vi "Task 4.vi"() -> ()   [LabVIEW 2025]
uses:
  <vilib>/httpClient/POSTBuffer.vi
  <vilib>/httpClient/LabVIEWHTTPClient.lvlib
panel:
  out "Corrected Text":string
  in  "Select correct word":string(combo)
  out "Error Text underlined":string
  in  "?":bool
  in  "User Input":string
  # "Users can check spelling inside a text box. Misspelled words are underlined, and users can select the correct suggestion to replace the incorrect word."
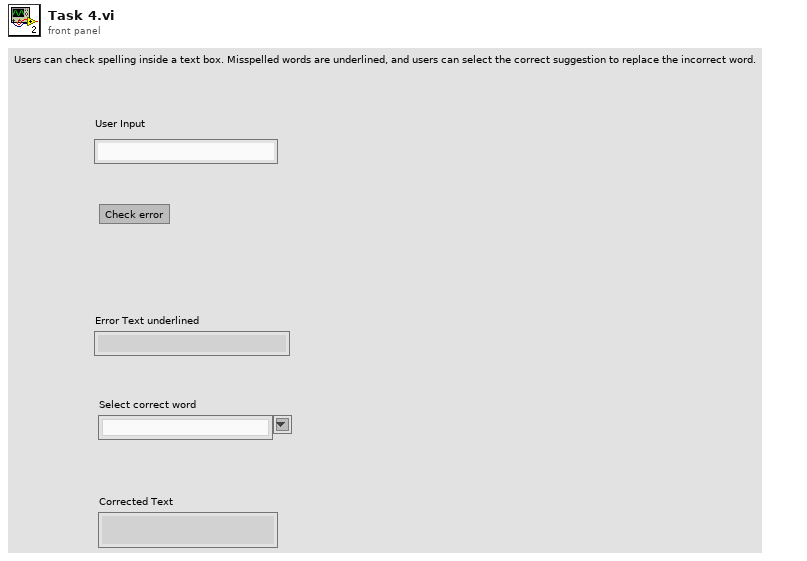
[diagram p1: front panel]
types:
  T1 = cluster{"matches":cluster{"offset":i32, "length":i32, "message":string, "replacements":cluster{"value":string}[]}[]}
  T2 = typedef "LabVIEWHTTPClient.lvlib/ClientHandle.ctl" = refnum<k1>
  T3 = cluster{"offset":i32, "length":i32, "message":string, "replacements":cluster{"value":string}[]}[]
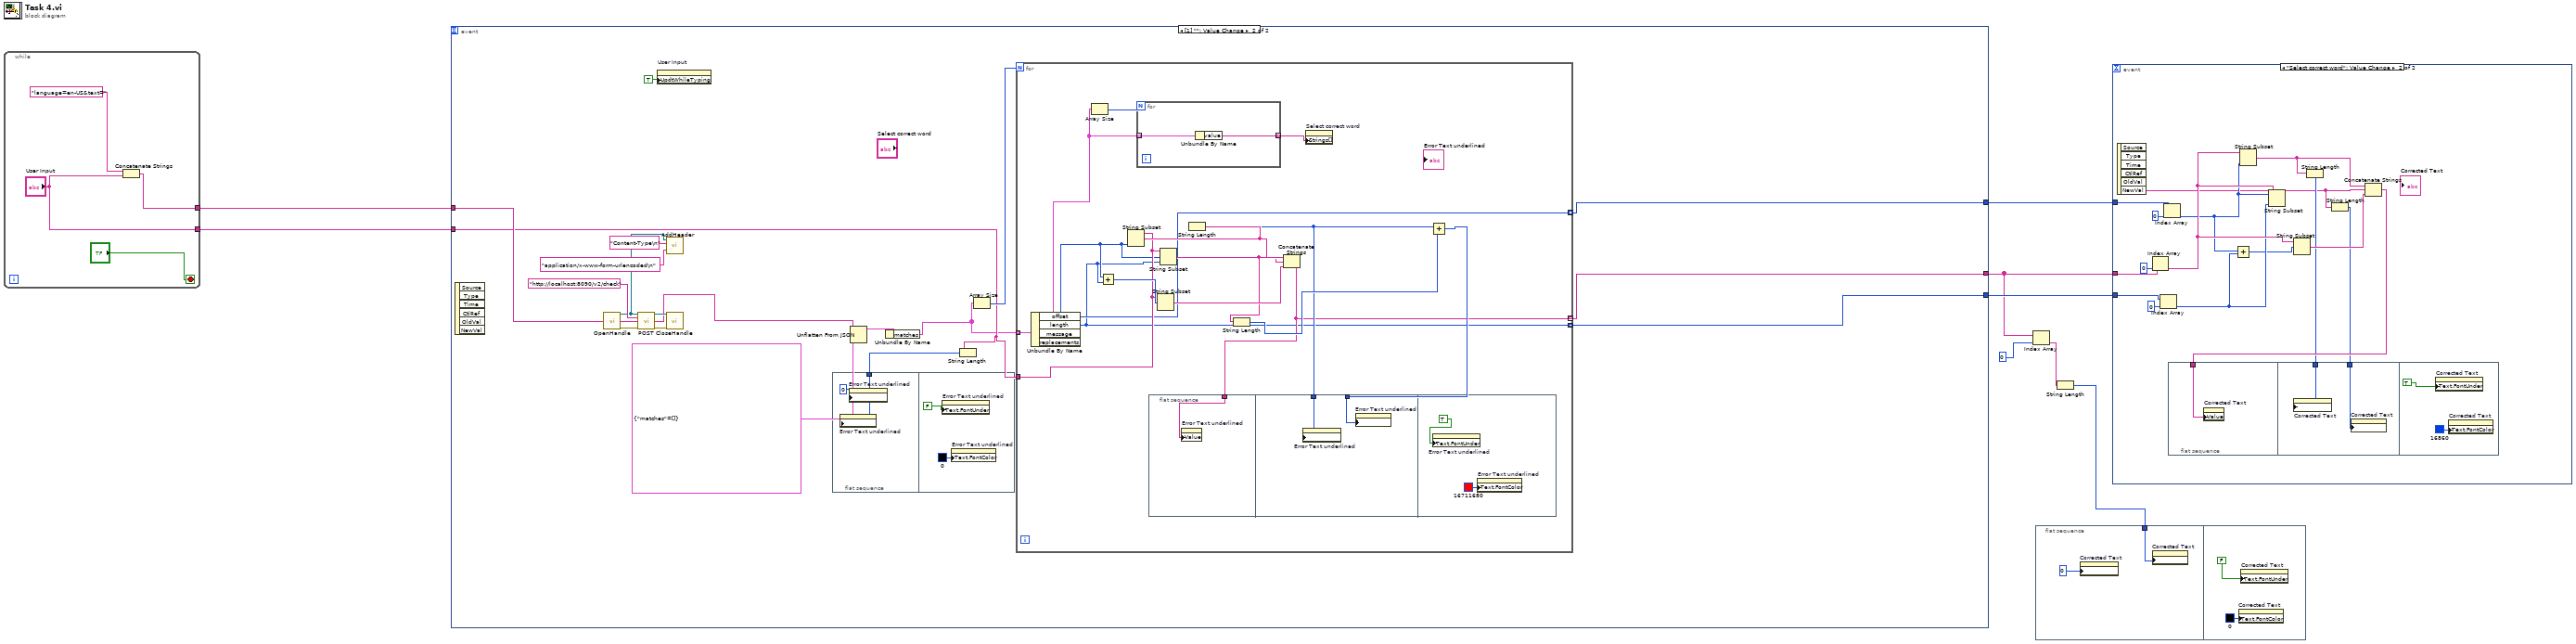
[diagram p0: block diagram]
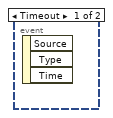
[diagram p2: hidden frame]
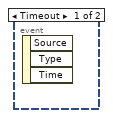
[diagram p3: hidden frame]
diagram:
  n1 = while {
    tunnel: ["User Input"] -> w2
    tunnel: [w10] -> w1
    stop <- "?" stop-if-true
    n2 = Concatenate Strings("language=en-US&text=", "User Input") -> (w10:string)
  }
  n3 = event shown="[1] \"\": Value Change" {
    selector: _ -> [_ _]
    dyn-events: _ -> [_ _]
    timeout: _ -> [_ _]
    tunnel: w1 -> [_ w24]
    tunnel: w2 -> [_ w19]
    tunnel: [_ w16] -> w8
    tunnel: [_ w15] -> w5
    tunnel: [_ w14] -> w7
    event Timeout {
      n4 = event-data() -> ()  [unwired: 1 in, 3 out]
    }
    event Value Change {
      n5 = event-data() -> ()  [unwired: 1 in, 6 out]
      n6 = call <vilib>:"OpenHandle.vi"() -> ("client handle out"=w27:T2, "error out"=w28:errorcluster)  [unwired: 14 in]
      n7 = call-poly <vilib>:"POST.vi"("client handle"=w27, "url"="http://localhost:8090/v2/check", "buffer"=w24, "error in (no error)"=w28) -> ("client handle out"=w30:T2, "body"=w23:string, "error out"=w29:errorcluster)  [unwired: 8 in, 1 out]
      n8 = property on="User Input" class="Str"("UpdtWhileTyping"=TRUE ("Update While Typing?")) -> ()  [unwired: 2 in, 2 out]
      n9 = call <vilib>:"AddHeader.vi"("client handle"=w27, "header"="Content-Type\n", "value"="application/x-www-form-urlencoded\n") -> ()  [unwired: 11 in, 2 out]
      n10 = call <vilib>:"CloseHandle.vi"("client handle"=w30, "error in (no error)"=w29) -> ()  [unwired: 13 in, 1 out]
      n11 = flat-sequence {
        tunnel: w18 -> [w32]
        frame #0 {
          n12 = property on="Error Text underlined" class="Str"("Text.Selection End"=w32) -> ()  [unwired: 2 in, 2 out]
          n13 = property on="Error Text underlined" class="Str"("Text.Selection Start"=u32 0 ("Text.Selection:Start")) -> ()  [unwired: 2 in, 2 out]
        }
        frame #1 {
          n14 = property on="Error Text underlined" class="Str"("Text.FontUnder"=FALSE) -> ()  [unwired: 2 in, 2 out]
          n15 = property on="Error Text underlined" class="Str"("Text.FontColor"=u32 0 ("Text.Font:Color")) -> ()  [unwired: 2 in, 2 out]
        }
      }
      n16 = Unflatten From JSON(JSON string=w23, type and defaults=T1 {"matches"=[]}) -> (value=w21:T1)  [unwired: 5 in, 1 out]
      n17 = Unbundle By Name(w21) -> ("matches"=w17:T3)
      n18 = String Length(string=w19) -> (length=w18:i32)
      n19 = Array Size(array=w17) -> (size(s)=w20:i32)
      n20 = for {
        N: w20 -> [_]
        tunnel: w17 -> [w50] mode=indexing
        tunnel: w19 -> [w42]
        tunnel: [w38] -> w16 mode=indexing
        tunnel: [w37] -> w15 mode=indexing
        tunnel: [w36] -> w14 mode=indexing
        n21 = Unbundle By Name(w50) -> ("offset"=w38:i32, "length"=w36:i32, "replacements"=w40:cluster{"value":string}[])  [unwired: 1 out]
        n22 = Array Size(array=w40) -> (size(s)=w41:i32)
        n23 = Add(x=w38, y=w36) -> (x+y=w49:i32)
        n24 = String Subset(string=w42, length (rest)=w38) -> (substring=w48:string)  [unwired: 1 in]
        n25 = for {
          N: w41 -> [_]
          tunnel: w40 -> [w52] mode=indexing
          tunnel: [w51] -> w39 mode=indexing
          n26 = Unbundle By Name(w52) -> ("value"=w51:string)
        }
        n27 = flat-sequence {
          tunnel: w37 -> [w53]
          tunnel: w43 -> [w55]
          tunnel: w44 -> [w54]
          frame #0 {
            n28 = property on="Error Text underlined" class="Str"("Value"=w53) -> ()  [unwired: 2 in, 2 out]
          }
          frame #1 {
            n29 = property on="Error Text underlined" class="Str"("Text.Selection Start"=w55) -> ()  [unwired: 2 in, 2 out]
            n30 = property on="Error Text underlined" class="Str"("Text.Selection End"=w54) -> ()  [unwired: 2 in, 2 out]
          }
          frame #2 {
            n31 = property on="Error Text underlined" class="Str"("Text.FontUnder"=TRUE) -> ()  [unwired: 2 in, 2 out]
            n32 = property on="Error Text underlined" class="Str"("Text.FontColor"=u32 16711680 ("Text.Font:Color")) -> ()  [unwired: 2 in, 2 out]
          }
        }
        n33 = String Subset(string=w42, offset (0)=w49) -> (substring=w47:string)  [unwired: 1 in]
        n34 = String Subset(string=w42, offset (0)=w38, length (rest)=w36) -> (substring=w46:string)
        n35 = String Length(string=w48) -> (length=w43:i32)
        n36 = String Length(string=w46) -> (length=w45:i32)
        n37 = Concatenate Strings(w48, w46, w47) -> (w37:string)
        n38 = property on="Select correct word" class="CmbBox"("Strings[]"=w39) -> ()  [unwired: 2 in, 2 out]
        n39 = Add(x=w43, y=w45) -> (x+y=w44:i32)
      }
    }
  }
  n40 = Index Array(array=w5, index=0) -> (element=w4:string)
  n41 = flat-sequence {
    tunnel: w3 -> [w59]
    frame #0 {
      n42 = property on="Corrected Text" class="Str"("Text.Selection Start"=0) -> ()  [unwired: 2 in, 2 out]
      n43 = property on="Corrected Text" class="Str"("Text.Selection End"=w59) -> ()  [unwired: 2 in, 2 out]
    }
    frame #1 {
      n44 = property on="Corrected Text" class="Str"("Text.FontColor"=u32 0 ("Text.Font:Color")) -> ()  [unwired: 2 in, 2 out]
      n45 = property on="Corrected Text" class="Str"("Text.FontUnder"=FALSE) -> ()  [unwired: 2 in, 2 out]
    }
  }
  n46 = String Length(string=w4) -> (length=w3:i32)
  n47 = event shown="[1] \"Select correct word\": Value Change" {
    selector: _ -> [_ _]
    dyn-events: _ -> [_ _]
    timeout: _ -> [_ _]
    tunnel: w8 -> [_ w77]
    tunnel: w5 -> [_ w74]
    tunnel: w7 -> [_ w71]
    event Timeout {
      n48 = event-data() -> ()  [unwired: 1 in, 3 out]
    }
    event "Select correct word": Value Change {
      n49 = event-data() -> ("NewVal"=w63:string)  [unwired: 1 in, 5 out]
      n50 = Index Array(array=w74, index=0) -> (element=w73:string)
      n51 = Index Array(array=w71, index=0) -> (element=w69:i32)
      n52 = Index Array(array=w77, index=0) -> (element=w70:i32)
      n53 = flat-sequence {
        tunnel: w66 -> [w78]
        tunnel: w64 -> [w80]
        tunnel: w62 -> [w79]
        frame #0 {
          n54 = property on="Corrected Text" class="Str"("Value"=w78) -> ()  [unwired: 2 in, 2 out]
        }
        frame #1 {
          n55 = property on="Corrected Text" class="Str"("Text.Selection Start"=w80) -> ()  [unwired: 2 in, 2 out]
          n56 = property on="Corrected Text" class="Str"("Text.Selection End"=w79) -> ()  [unwired: 2 in, 2 out]
        }
        frame #2 {
          n57 = property on="Corrected Text" class="Str"("Text.FontUnder"=TRUE) -> ()  [unwired: 2 in, 2 out]
          n58 = property on="Corrected Text" class="Str"("Text.FontColor"=u32 16860 ("Text.Font:Color")) -> ()  [unwired: 2 in, 2 out]
        }
      }
      n59 = Add(x=w70, y=w69) -> (x+y=w68:i32)
      n60 = String Subset(string=w73, length (rest)=w70) -> (substring=w65:string)  [unwired: 1 in]
      n61 = String Subset(string=w73, offset (0)=w70, length (rest)=w69) -> ()  [unwired: 1 out]
      n62 = String Subset(string=w73, offset (0)=w68) -> (substring=w67:string)  [unwired: 1 in]
      n63 = String Length(string=w65) -> (length=w64:i32)
      n64 = String Length(string=w63) -> (length=w62:i32)
      n65 = Concatenate Strings(w65, w63, w67) -> (w66:string)
    }
  }
